vi "Auto Inspection_TraySet.vi"(0 "TableIn":string[][](array[string])=[["Default", "", "", " 0"], ["Case1", "", "", "1"], ["Case2", "", "", "2"], ["Case3", "", "", "3"], ["Case4", "", "", "4"], ["Case5", "", "", "5"], ["Case6", "", "", "6"], ["Case7", "", "", "7"], ["Case8", "", "", "8"], ["Case9", "", "", "9"], ["Case10", "", "", "10"], ["", "", "", ""], ["", "", "", ""], ["", "", "", ""], ["", "", "", ""], ["", "", "", ""], ["", "", "", ""], ["", "", "", ""], ["", "", "", ""], ["", "", "", ""], ["", "", "", ""], ["22", "", "", ""], ["23", "", "", ""], ["24", "", "", ""], ["25", "", "", ""]], 1 "Action":T2(ring)=enum."WrteAll", 5 "X":i32, 7 "Y":i32, 9 "DataIn":string, 11 "error in":errorcluster, 12 "Name":T1) -> (4 "LSTableOut":string[][](array[string]), 6 "AITableOut":string[][](array[string]), 8 "LSMap":string[][](array[string]), 10 "DataOut":string, 14 "AIMap":string[][](array[string]), 15 "error out":errorcluster)   [LabVIEW 2019]
uses:
  Auto Inspection Tray Map Name.ctl
  09bdc40f-24f8-42fa-be14-94a5734f4f81.vi
  3a88f7dc-0fdf-4cec-95e5-a4f3429e1c34.vi
  LLB/Commonly VI/Main Glb.vi
  <vilib>/JDP Science/JSONtext/Variant to JSON Text.vi
  <vilib>/JDP Science/JSONtext/JSON text to Variant.vi
  LLB/Commonly VI.lvlib
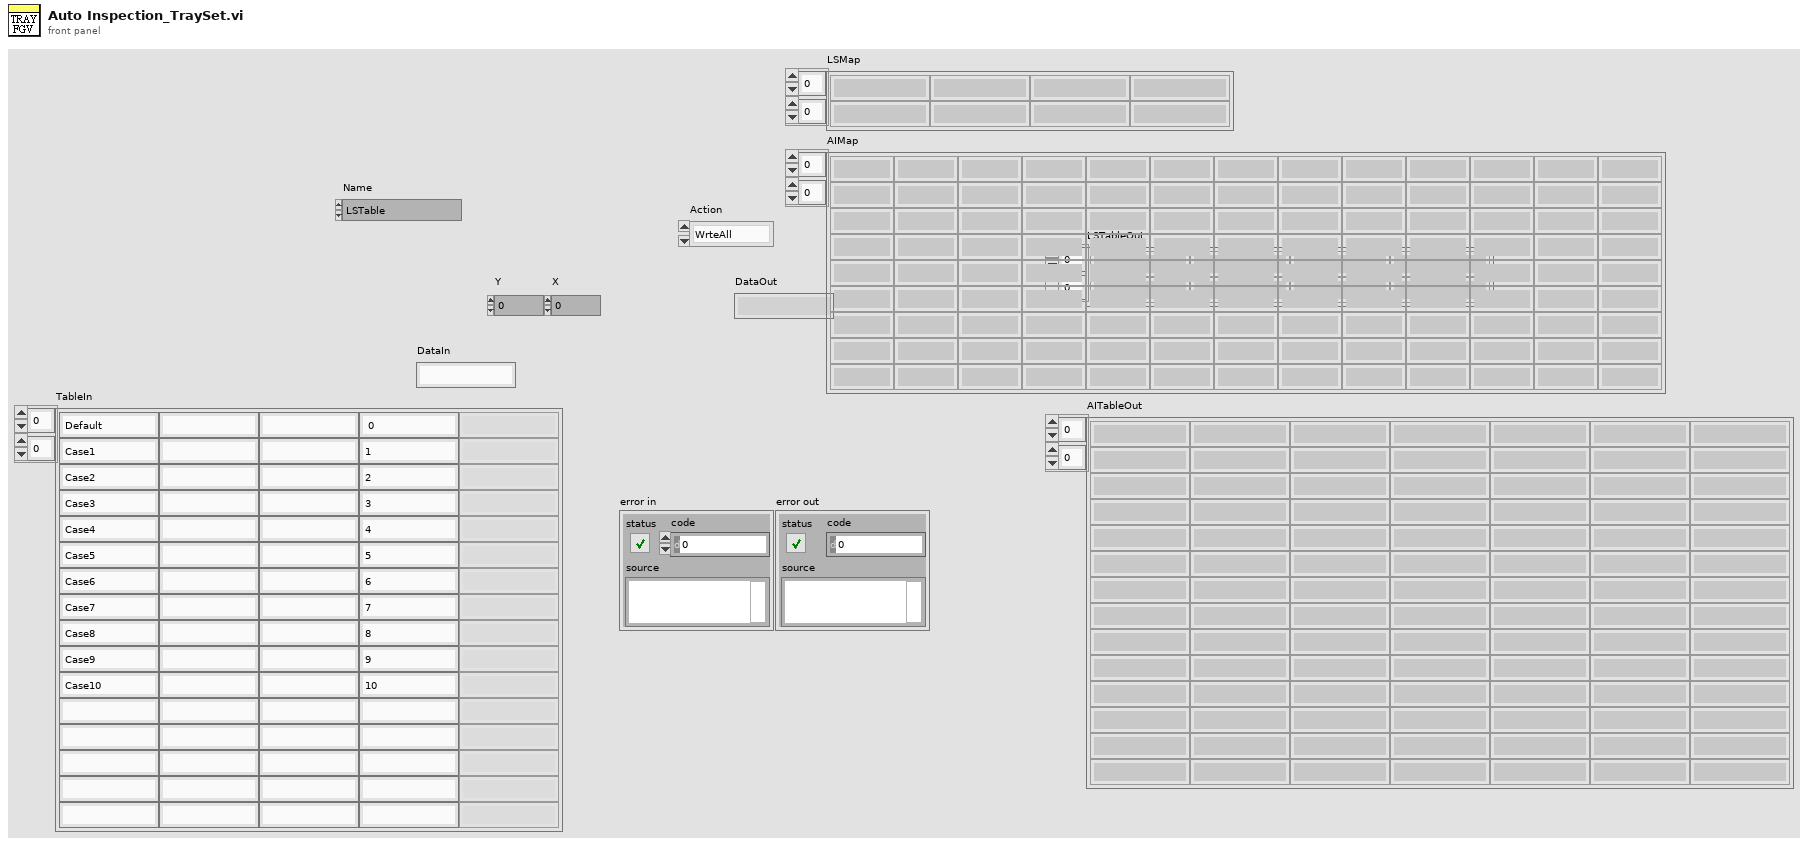
[diagram p1: front panel]
types:
  T1 = typedef "Auto Inspection Tray Map Name.ctl" = enum16{"LSTable", "AITable", "LSMap", "AIMap"}
  T2 = enum16{"Initial", "Write", "Read", "Save", "Load", "WrteAll"}
  T3 = cluster{"LSTableOut":string[][], "AITableOut":string[][], "LSMap":string[][], "AIMap":string[][]}
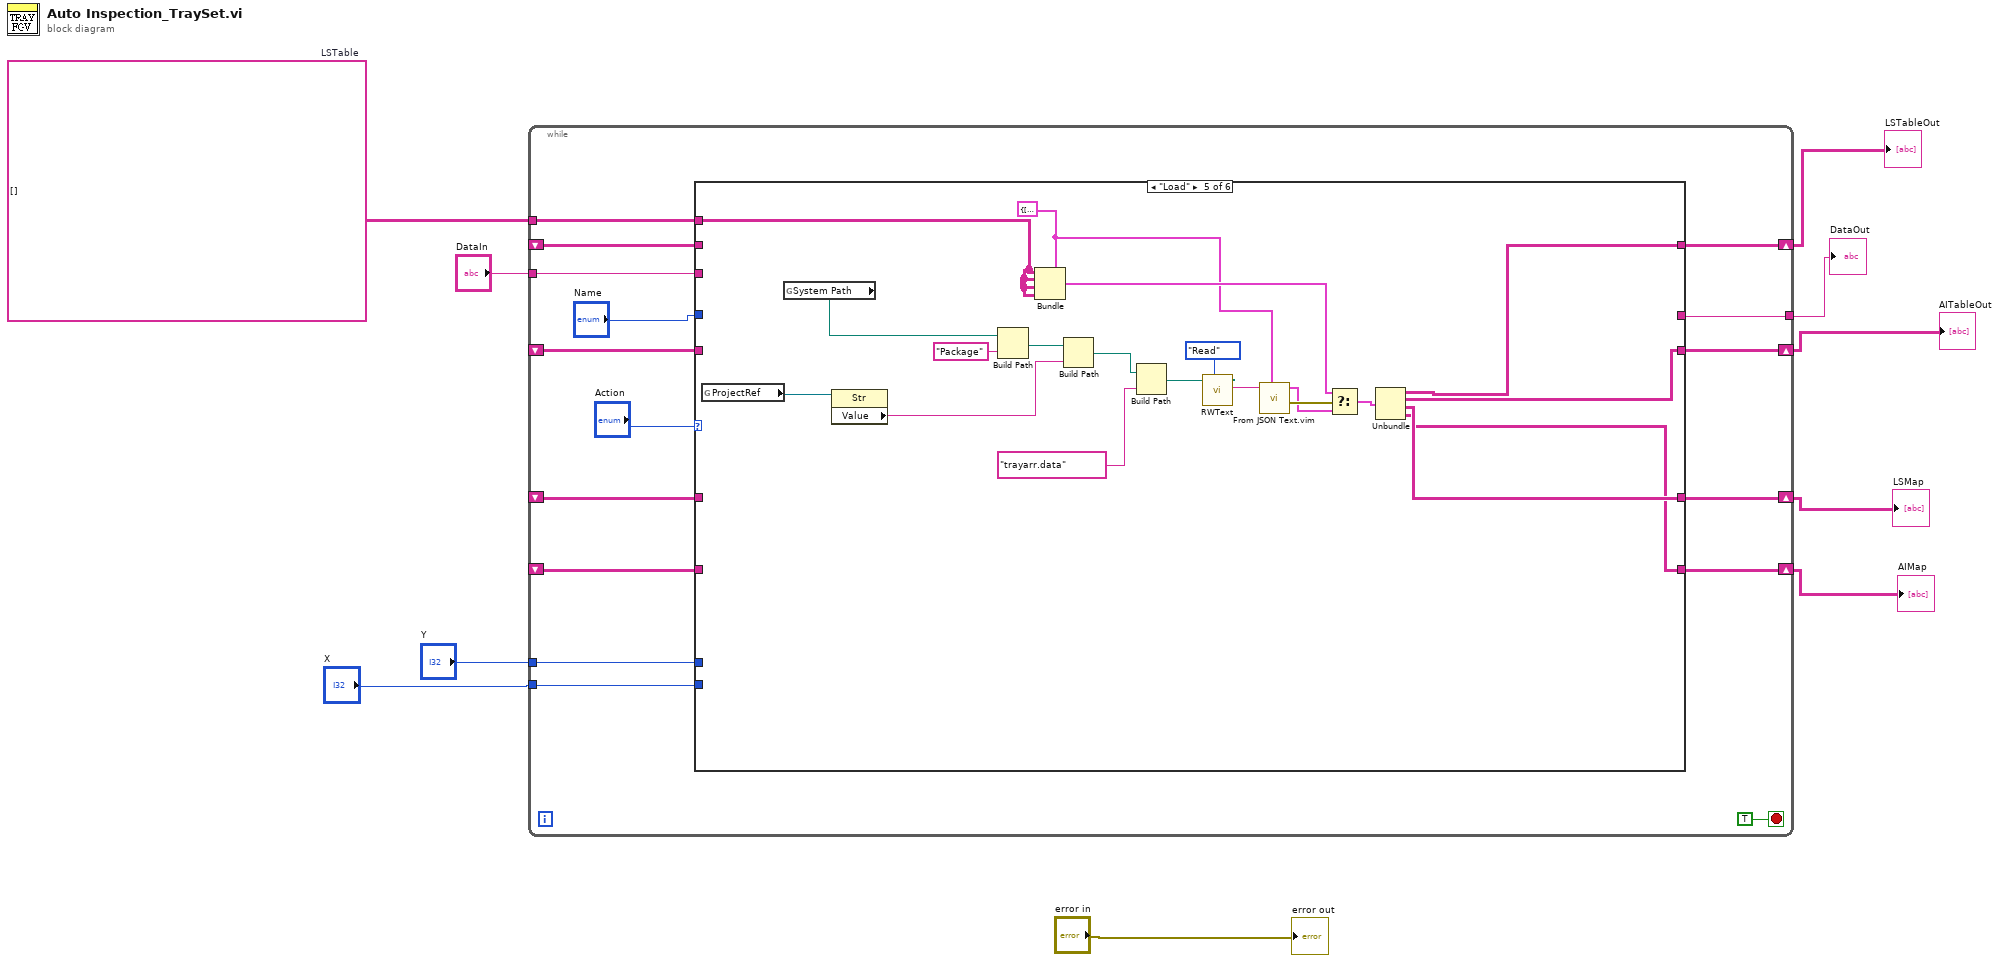
[diagram p0: block diagram]
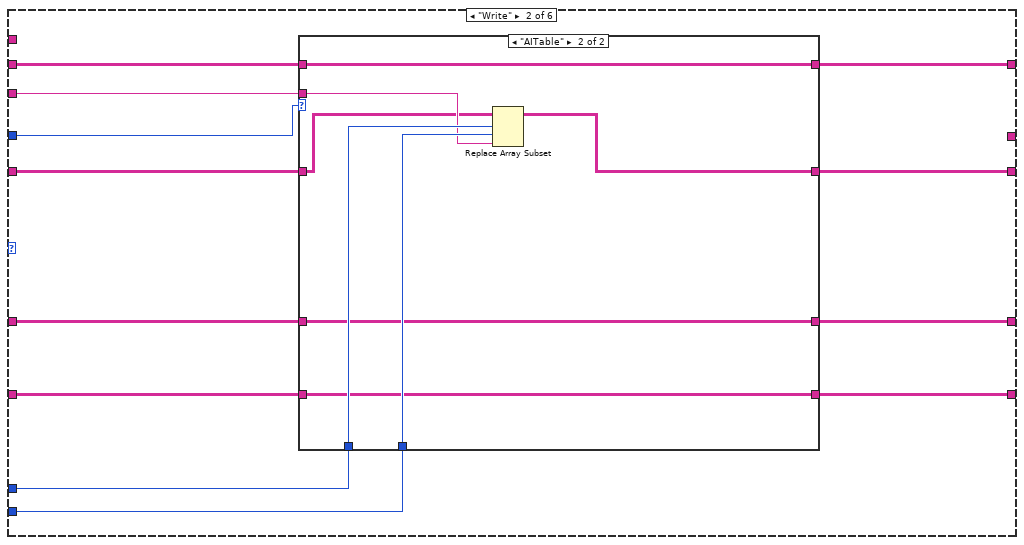
[diagram p3: hidden frame]
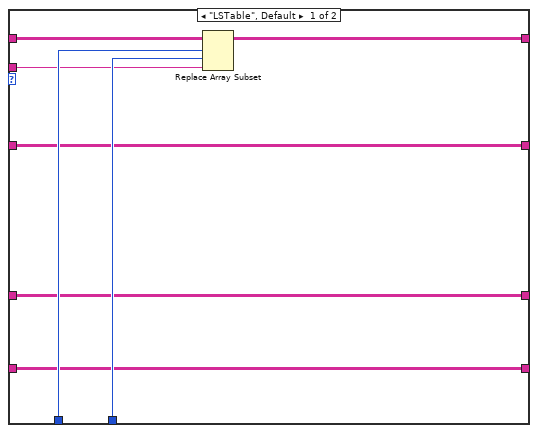
[diagram p4: hidden frame]
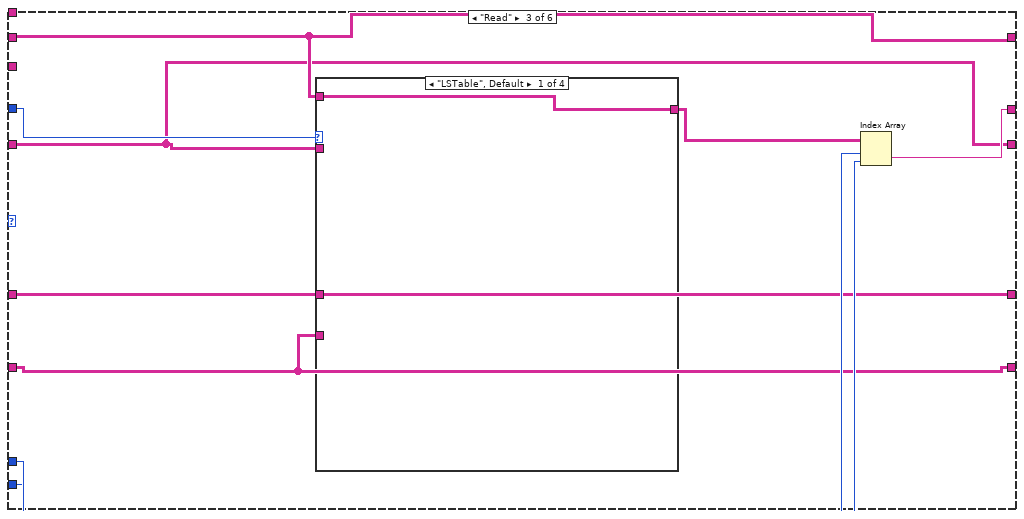
[diagram p5: hidden frame]
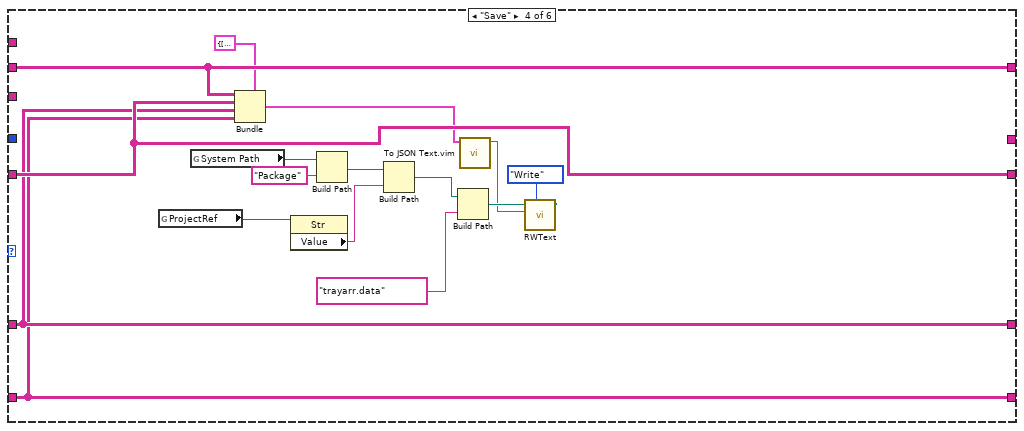
[diagram p9: hidden frame]
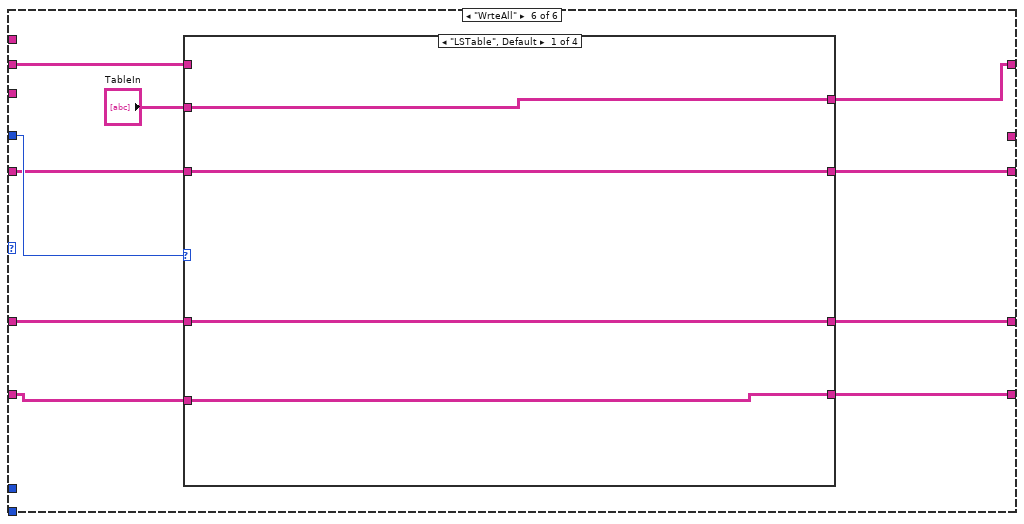
[diagram p10: hidden frame]
diagram:
  w7 = string[][] []  # LSTable
  n1 = while {
    shift-right: [w26] -> w6
    shift-left: _ -> [w25]
    tunnel: w7 -> [w24]
    tunnel: "X" -> [w22]
    tunnel: "Y" -> [w21]
    tunnel: "DataIn" -> [w20]
    shift-right: [w18] -> w4
    shift-left: _ -> [w17]
    shift-right: [w15] -> w3
    shift-left: _ -> [w13]
    shift-right: [w14] -> w2
    shift-left: _ -> [w12]
    tunnel: [w11] -> w1
    stop <- TRUE stop-if-true
    n2 = case shown="\"Load\"" "Action" {
      tunnel: [w27 w39 w64 w74 w93 w113] -> w26
      tunnel: w25 -> [_ w38 w64 w74 _ w105]
      tunnel: w24 -> [w27 _ _ _ w87 _]
      tunnel: w22 -> [_ w37 w60 _ _ _]
      tunnel: w21 -> [_ w36 w62 _ _ _]
      tunnel: w20 -> [_ w35 _ _ _ _]
      tunnel: [w27 w32 w58 w73 w92 w110] -> w18
      tunnel: w17 -> [_ w33 w58 w73 _ w111]
      tunnel: "Name" -> [_ w34 w63 _ _ w114]
      tunnel: [w27 w29 w57 w70 w86 w109] -> w15
      tunnel: [w27 w28 w56 w69 w85 w106] -> w14
      tunnel: w13 -> [_ w31 w57 w70 _ w108]
      tunnel: w12 -> [_ w30 w56 w69 _ w107]
      tunnel: [_ _ w61 _ _ _] -> w11
      frame "Initial", Default {
      }
      frame "Write" {
        n3 = case shown="\"AITable\"" w34 {
          tunnel: [w47 w50] -> w39
          tunnel: w38 -> [w46 w50]
          tunnel: w37 -> [w45 w55]
          tunnel: w36 -> [w44 w54]
          tunnel: w35 -> [w43 w53]
          tunnel: w33 -> [w42 w51]
          tunnel: [w42 w52] -> w32
          tunnel: w31 -> [w41 w49]
          tunnel: w30 -> [w40 w48]
          tunnel: [w41 w49] -> w29
          tunnel: [w40 w48] -> w28
          frame "LSTable", Default {
            n4 = Replace Array Subset(array=w46, new element=w43, index (row)=w44, index (col)=w45) -> (w47:string[][])
          }
          frame "AITable" {
            n5 = Replace Array Subset(array=w51, new element=w53, index (row)=w54, index (col)=w55) -> (w52:string[][])
          }
        }
      }
      frame "Read" {
        n6 = case shown="\"LSTable\", Default" w63 {
          tunnel: w64 -> [w65 _ _ _]
          tunnel: [w65 w66 w67 w68] -> w59
          tunnel: w58 -> [_ w66 _ _]
          tunnel: w57 -> [_ _ w67 _]
          tunnel: w56 -> [_ _ _ w68]
          frame "LSTable", Default {
          }
          frame "AITable" {
          }
          frame "LSMap" {
          }
          frame "AIMap" {
          }
        }
        n7 = Index Array(array=w59, index (row)=w62, index (col)=w60) -> (element=w61:string)
      }
      frame "Save" {
        n8 = global read "Main Glb.vi" "ProjectRef"() -> (w81:refnum<vi>)
        n9 = global read "Main Glb.vi" "System Path"() -> (w84:path)
        n10 = Bundle(cluster=T3 {"LSTableOut"=[], "AITableOut"=[], "LSMap"=[], "AIMap"=[]}, "LSTableOut"=w74, "AITableOut"=w73, "LSMap"=w70, "AIMap"=w69) -> (w72:T3)
        n11 = property class="Str"(reference=w81) -> ("Value"=w80:string)  [unwired: 1 in, 2 out]
        n12 = Build Path(base path=w84, name or relative path="Package") -> (appended path=w82:path)
        n13 = Build Path(base path=w82, name or relative path=w80) -> (appended path=w78:path)
        n14 = Build Path(base path=w78, name or relative path="trayarr.data") -> (appended path=w76:path)
        n15 = call "To JSON Text.vim"("Anything"=w72) -> ("<JSON>"=w75:string)  [unwired: 9 in, 1 out]
        n16 = call "RWText.vi"("Action"=enum16{"Read", "Write"}."Write", "TextIn"=w75, "file path (use dialog)"=w76) -> ()  [unwired: 7 in, 2 out]
      }
      frame "Load" {
        w88 = T3 {"LSTableOut"=[], "AITableOut"=[], "LSMap"=[], "AIMap"=[]}
        n17 = global read "Main Glb.vi" "ProjectRef"() -> (w101:refnum<vi>)
        n18 = global read "Main Glb.vi" "System Path"() -> (w104:path)
        n19 = property class="Str"(reference=w101) -> ("Value"=w100:string)  [unwired: 1 in, 2 out]
        n20 = Build Path(base path=w104, name or relative path="Package") -> (appended path=w102:path)
        n21 = Bundle(cluster=w88, "LSTableOut"=w87, "AITableOut"=w87, "LSMap"=w87, "AIMap"=w87) -> (w89:T3)
        n22 = Build Path(base path=w102, name or relative path=w100) -> (appended path=w98:path)
        n23 = Build Path(base path=w98, name or relative path="trayarr.data") -> (appended path=w96:path)
        n24 = call "RWText.vi"("Action"=enum16{"Read", "Write"}."Read", "file path (use dialog)"=w96) -> ("textOut"=w95:string)  [unwired: 8 in, 1 out]
        n25 = call "From JSON Text.vim"("Data Type and Default Value"=w88, "JSON"=w95) -> ("error out"=w91:errorcluster, "Data out"=w90:T3)  [unwired: 8 in]
        n26 = Select(t=w89, s=w91, f=w90) -> (s? t:f=w94:T3)
        n27 = Unbundle(w94) -> ("LSTableOut"=w93:string[][], "AITableOut"=w92:string[][], "LSMap"=w86:string[][], "AIMap"=w85:string[][])
      }
      frame "WrteAll" {
        n28 = case shown="\"LSTable\", Default" w114 {
          tunnel: [w118 w120 w125 w130] -> w113
          tunnel: "TableIn" -> [w118 w119 w123 w127]
          tunnel: w111 -> [w117 _ w124 w129]
          tunnel: [w117 w119 w124 w129] -> w110
          tunnel: [w116 w122 w123 w128] -> w109
          tunnel: w108 -> [w116 w122 _ w128]
          tunnel: w107 -> [w115 w121 w126 _]
          tunnel: [w115 w121 w126 w127] -> w106
          tunnel: w105 -> [_ w120 w125 w130]
          frame "LSTable", Default {
          }
          frame "AITable" {
          }
          frame "LSMap" {
          }
          frame "AIMap" {
          }
        }
      }
    }
  }
  "DataOut" <- w1
  "LSTableOut" <- w6
  "AITableOut" <- w4
  "LSMap" <- w3
  "AIMap" <- w2
  "error out" <- "error in"
